vi "Main -- single image.vi"() -> ()   [LabVIEW 2013]
uses:
  <vilib>/userdefined/High Color/IMAQdx.ctl
  <vilib>/vision/driver/NI_Vision_Acquisition_Software.lvlib
  <vilib>/vision/NI_Vision_Development_Module.lvlib
panel:
  in  "webcam":T1="cam0"
  in  "Filter Parameters":T2={"Sigma"=1.0, "HThresh"=0.9, "LThres"=0.2, "WindowSize"=9} {"LThres" min=0 max=1 format="%.2f"; "HThresh" min=0 max=1 format="%.2f"; "Sigma" min=0 max=1 format="%.2f"}
  out "edges":T3(plugin-control)
  out "original":T3(plugin-control)
  # "LED Matrix demo"
  # "Webcam demo - single image"
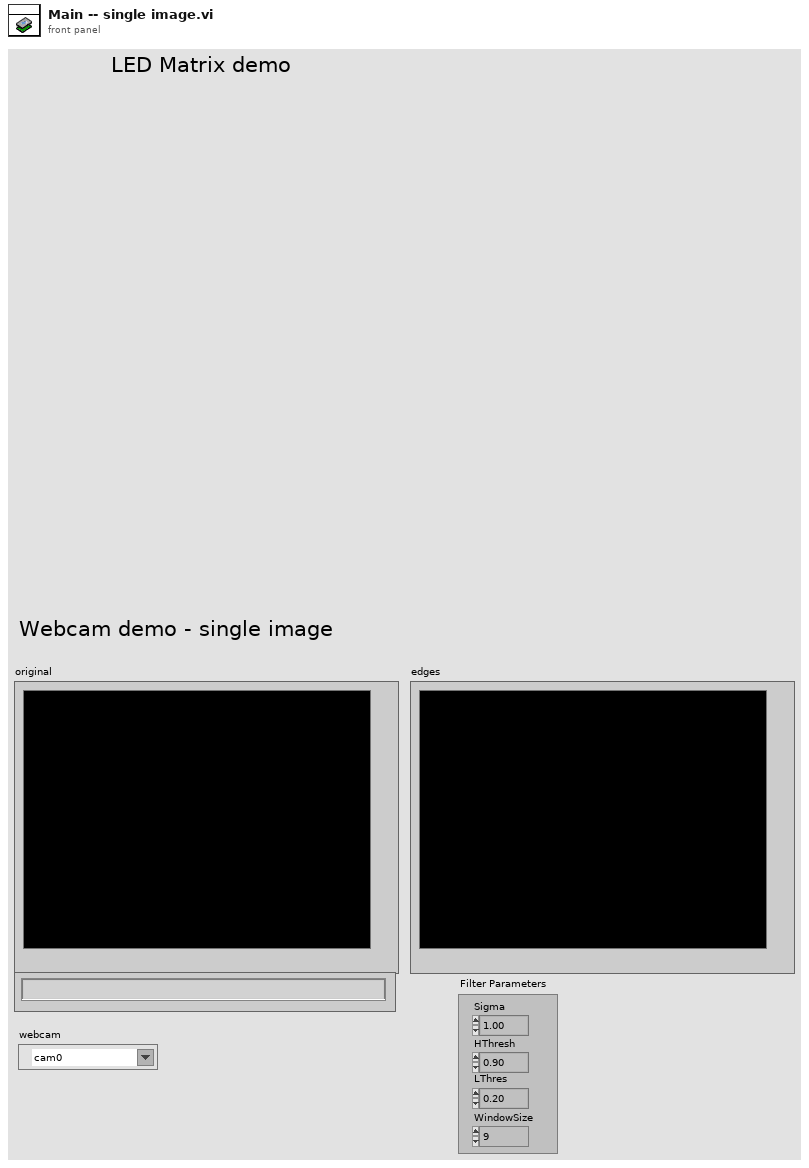
[diagram p1: front panel]
types:
  T1 = typedef "IMAQdx.ctl" = refnum<k21>
  T2 = cluster{"Sigma":sgl, "HThresh":sgl, "LThres":sgl, "WindowSize":i32}
  T3 = typedef "IMAQ Image.ctl" = refnum<image>
  T4 = typedef "Image Type" = u32
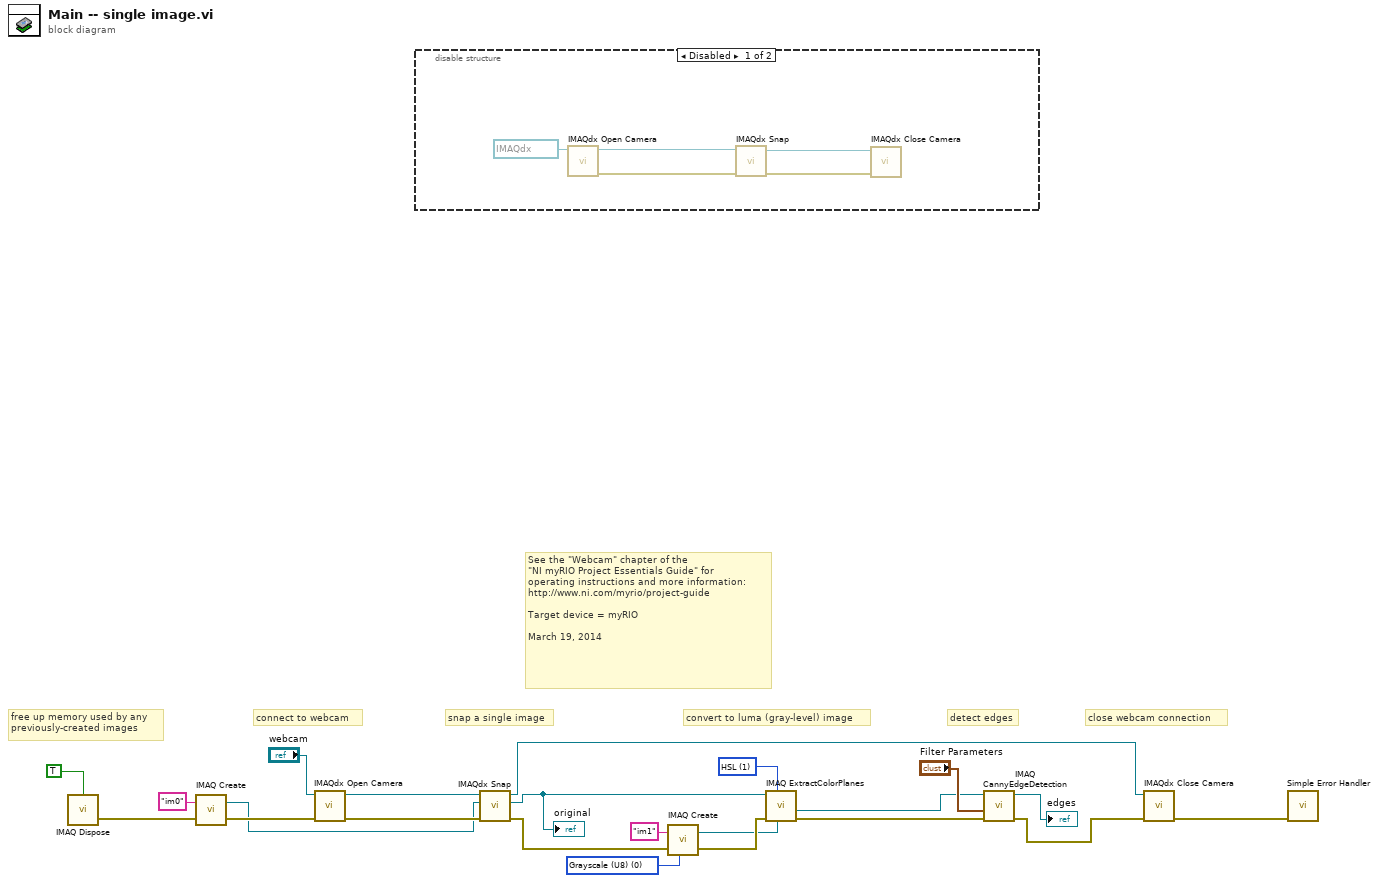
[diagram p0: block diagram]
diagram:
  w16 = T4 0 items=["Grayscale (U8)", "Grayscale (I16)", "Grayscale (SGL)", "Complex (CSG)", "RGB (U32)", "HSL (U32)", "RGB (U64)", "Grayscale (U16)"] ("Image Type")
  w20 = u16 1 items=["RGB", "HSL", "HSV", "HSI"] ("Color Mode")
  # "See the \"Webcam\" chapter of the\n\"NI myRIO Project Essentials Guide\" for\noperating instructions and more information: \nhttp://www.ni.com/myrio/project-guide\n\nTarget device = myRIO\n\nMarch 19, 2014"
  # "close webcam connection"
  # "connect to webcam"
  # "free up memory used by any\npreviously-created images"
  # "snap a single image"
  # "detect edges"
  # "convert to luma (gray-level) image"
  n1 = call "IMAQ Dispose"("All Images? (No)"=TRUE) -> ("error out"=w9:errorcluster)  [unwired: 5 in]
  n2 = call "IMAQ Create"("Image Name"="im0", "error in (no error)"=w9) -> ("New Image"=w4:T3, "error out"=w8:errorcluster)  [unwired: 2 in, 1 out]
  n3 = call <vilib>:"IMAQdx Open Camera.vi"("error in"=w8, "Session In"="webcam") -> ("error out"=w7:errorcluster, "Session Out"=w5:T1)  [unwired: 8 in]
  n4 = disable-structure shown="Disabled" {
    frame Disabled {
      n5 = call <vilib>:"IMAQdx Open Camera.vi"("Session In"=T1 "cam0") -> ("error out"=w26:errorcluster, "Session Out"=w25:T1)  [unwired: 9 in]
      n6 = call <vilib>:"IMAQdx Snap.vi"("error in"=w26, "Session In"=w25) -> ("error out"=w24:errorcluster, "Session Out"=w23:T1)  [unwired: 7 in, 1 out]
      n7 = call <vilib>:"IMAQdx Close Camera.vi"("error in"=w24, "Session In"=w23) -> ()  [unwired: 9 in, 1 out]
    }
    frame Enabled {
    }
  }
  n8 = call <vilib>:"IMAQdx Snap.vi"("error in"=w7, "Image In"=w4, "Session In"=w5) -> ("error out"=w15:errorcluster, "Image Out"=w13:T3, "Session Out"=w1:T1)  [unwired: 6 out]
  "original" <- w13
  n9 = call "IMAQ Create"("Image Name"="im1", "Image Type"=w16, "error in (no error)"=w15) -> ("New Image"=w11:T3, "error out"=w14:errorcluster)  [unwired: 1 in, 1 out]
  n10 = call "IMAQ ExtractColorPlanes"("Blue or Luma or Val or Inten Plane"=w11, "Color Mode"=w20, "error in (no error)"=w14, "Image Src"=w13) -> ("error out"=w17:errorcluster, "Blue or Luma or Val or Inten Plane out"=w18:T3)  [unwired: 4 in, 2 out]
  n11 = call "IMAQ CannyEdgeDetection"("Image Src"=w18, "Filter Parameters"="Filter Parameters", "error in (no error)"=w17) -> ("Image Dst Out"=→"edges":T3, "error out"=w2:errorcluster)  [unwired: 5 in]
  n12 = call <vilib>:"IMAQdx Close Camera.vi"("error in"=w2, "Session In"=w1) -> ("error out"=w3:errorcluster)  [unwired: 9 in]
  n13 = call <vilib>:"Simple Error Handler.vi"("error in (no error)"=w3) -> ()  [unwired: 4 in, 5 out]
